vi "degreestopos.vi"(3 "Degrees @ Home (15.00)":dbl=15.0 format="%.2f", 4 "Ticks per degree (28571.43)":dbl=28571.43 format="%.2f", 5 "Degrees":dbl=10.0 min=8.0 max=70.0 format="%.2f") -> (1 "Position":i32)   [LabVIEW 2015]
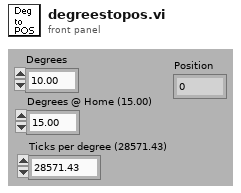
[diagram p1: front panel]
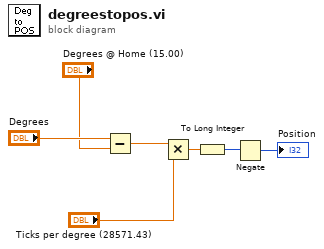
[diagram p0: block diagram]
diagram:
  n1 = Subtract(x="Degrees", y="Degrees @ Home (15.00)") -> (x-y=w6:dbl)
  n2 = Multiply(x=w6, y="Ticks per degree (28571.43)") -> (x*y=w5:dbl)
  n3 = To Long Integer(number=w5) -> (32bit integer=w3:i32)
  n4 = Negate(x=w3) -> (-x=→"Position":i32)
